vi "Periodic Tasks.vi"(8 "error in":errorcluster) -> ()   [LabVIEW 2018]
doc: "This VI runs in parallel to other tasks. It can contain as many user-defined periodic loops as you need. These can carry out PID or other sorts of timed response."
uses:
  <vilib>/Rock Robotics/WPI/Solenoid/WPI_SolenoidValue.ctl
  Phoenix-LabVIEW/Motor Controller/Controls/CTRE_Phoenix_MotorControl_ControlMode.ctl
  <vilib>/Rock Robotics/WPI/Utilities/WPI_GetSetVariantRefNum.vi
  <vilib>/Rock Robotics/WPI/Solenoid/WPI_SolenoidSetEnum.vi
  Global 1.vi
  <vilib>/Rock Robotics/Network Tables/NT Write Boolean.vi
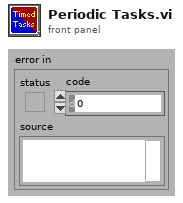
[diagram p1: front panel]
types:
  T1 = typedef "WPI_JoystickDevRef.ctl" = cluster{"Device":T2}
  T2 = typedef "WPI_JoystickDeviceEnum.ctl" = enum16{"USB 0", "USB 1", "USB 2", "USB 3", "USB 4", "USB 5"}
  T3 = typedef "WPI_RobotDriveDevRef.ctl" = cluster{"DevStatus":errorcluster, "Motors[]":T4[], "Square Inputs":bool, "Max Output":dbl}
  T4 = typedef "WPI_MotorControlDeviceRef.ctl" = cluster{"DeviceStatus":errorcluster, "Type":T5, "PWM":cluster{"PWM Channel":T6, "DeadBand":T7}, "CAN":cluster{"Device Number":u8, "SetOutput VI Ref":variant, "GetOutput VI Ref":variant, "Enable VI Ref":variant, "Disable VI Ref":variant, "Data":variant}, "Invert":bool, "DIO PWM":cluster{"PWM \"Enable\" Channel":T6, "DIOChannel":T8, "PWM Rate":dbl}}
  T5 = typedef "WPI_MotorControlType.ctl" = enum16{"PWM", "CAN", "DIO PWM"}
  T6 = typedef "FPGA_DIOPWMChannel.ctl" = enum8{"PWM 0", "PWM 1", "PWM 2", "PWM 3", "PWM 4", "PWM 5", "PWM 6", "PWM 7", "PWM 8", "PWM 9", "PWM MXP 0", "PWM MXP 1", "PWM MXP 2", "PWM MXP 3", "PWM MXP 4", "PWM MXP 5", "PWM MXP 6", "PWM MXP 7", "PWM MXP 8", "PWM MXP 9", "Invalid"}
  T7 = typedef "WPI_PWMDeadband.ctl" = cluster{"Name":string, "maxPositivePwm":i32, "minPositivePwm":i32, "centerPwm":i32, "maxNegativePwm":i32, "minNegativePwm":i32, "angularRange":u16}
  T8 = typedef "FPGA_DIOChannel.ctl" = enum8{"DIO 0", "DIO 1", "DIO 2", "DIO 3", "DIO 4", "DIO 5", "DIO 6", "DIO 7", "DIO 8", "DIO 9", "DIO MXP 0", "DIO MXP 1", "DIO MXP 2", "DIO MXP 3", "DIO MXP 4", "DIO MXP 5", "DIO MXP 6", "DIO MXP 7", "DIO MXP 8", "DIO MXP 9", "DIO MXP 10", "DIO MXP 11", "DIO MXP 12", "DIO MXP 13", "DIO MXP 14", "DIO MXP 15", "SPI Port CS1", "SPI Port CS2", "SPI Port CS3", "SPI Port MISO", "SPI Port MOSI", "Invalid"}
  T9 = cluster{"JoystickDevRef":T1, "RobotDriveDevRef":T3}
  T10 = typedef "WPI_SolenoidDevRef.ctl" = cluster{"DevStatus":errorcluster, "Pneumatics Control Module":u8, "Forward Solenoid Channel":T11, "Reverse Solenoid Channel":T11}
  T11 = typedef "WPI_SolenoidChannel.ctl" = enum8{"Solenoid 0", "Solenoid 1", "Solenoid 2", "Solenoid 3", "Solenoid 4", "Solenoid 5", "Solenoid 6", "Solenoid 7", "Invalid"}
  T12 = typedef "WPI_SolenoidValue.ctl" = enum16{"Off", "On", "Forward", "Reverse"}
  T13 = typedef "WPI_SwitchDevRef.ctl" = cluster{"DevStatus":errorcluster, "DIO Channel":T8, "CntIndex":T14, "Normally Closed":bool}
  T14 = typedef "FPGA_CounterCtrSystemIndex.ctl" = enum8{"Ctr 0", "Ctr 1", "Ctr 2", "Ctr 3", "Ctr 4", "Ctr 5", "Ctr 6", "Ctr 7", "Invalid"}
  T15 = typedef "CTRE_Phoenix_MotorControl_ControlMode.ctl" = u16
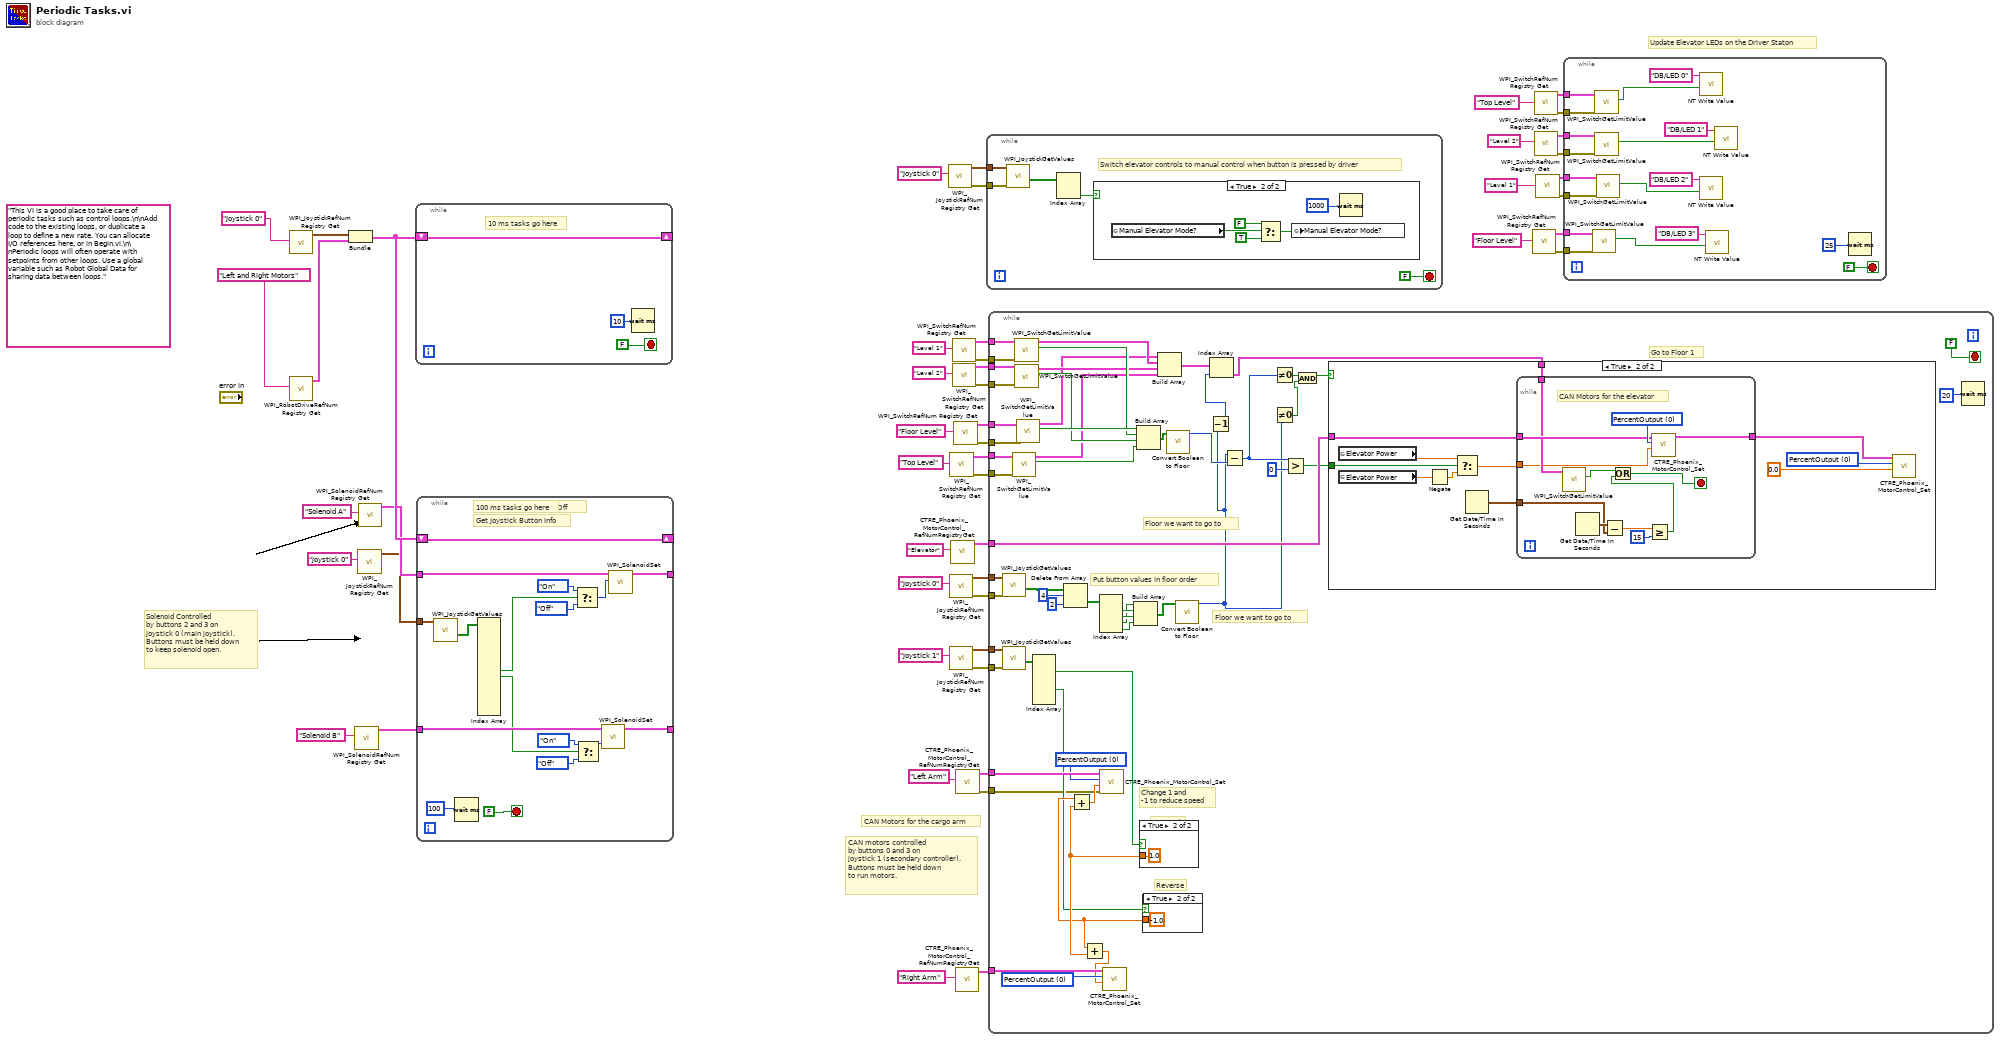
[diagram p0: block diagram]
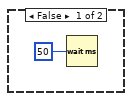
[diagram p2: hidden frame]
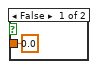
[diagram p3: hidden frame]
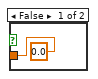
[diagram p4: hidden frame]
diagram:
  (unwired) "This VI is a good place to take care of periodic tasks such as control loops.\n\nAdd code to the existing loops, or duplicate a loop to define a new rate. You can allocate I/O references here, or in Begin.vi.\n\nPeriodic loops will often operate with setpoints from other loops. Use a global variable such as Robot Global Data for sharing data between loops."
  # "Update Elevator LEDs on the Driver Staton"
  # "CAN Motors for the cargo arm"
  # "CAN motors controlled\nby buttons 0 and 3 on \njoystick 1 (secondary controller).\nButtons must be held down\nto run motors."
  # "Solenoid Controlled\nby buttons 2 and 3 on \njoystick 0 (main joystick).\nButtons must be held down\nto keep solenoid open."
  n1 = call <vilib>:"WPI_JoystickRefNum Registry Get.vi"("refnum name"="Joystick 0") -> ("JoystickDevRef"=w49:T1)  [unwired: 1 in, 9 out]
  n2 = call <vilib>:"WPI_RobotDriveRefNum Registry Get.vi"("refnum name"="Left and Right Motors") -> ("RobotDriveDevRef"=w48:T3)  [unwired: 1 in, 9 out]
  n3 = Bundle("JoystickDevRef"=w49, "RobotDriveDevRef"=w48) -> (w47:T9)  [unwired: 1 out]
  n4 = call <vilib>:"WPI_SolenoidRefNum Registry Get.vi"("refnum name"="Solenoid B") -> ("SolenoidDevRef"=w39:T10)  [unwired: 9 in, 1 out]
  n5 = call <vilib>:"WPI_JoystickRefNum Registry Get.vi"("refnum name"="Joystick 0") -> ("JoystickDevRef"=w36:T1)  [unwired: 9 in, 1 out]
  n6 = call <vilib>:"WPI_SolenoidRefNum Registry Get.vi"("refnum name"="Solenoid A") -> ("SolenoidDevRef"=w40:T10)  [unwired: 9 in, 1 out]
  n7 = while {
    shift-right: [w52] -> _
    shift-left: w47 -> [w52]
    stop <- FALSE stop-if-true
    # "10 ms tasks go here"
    n8 = Wait (ms)(milliseconds to wait=u32 10) -> ()  [unwired: 1 out]
  }
  n9 = while {
    shift-right: [w69] -> _
    shift-left: w47 -> [w69]
    tunnel: w40 -> [w62]
    tunnel: w39 -> [w61]
    tunnel: [w60] -> _
    tunnel: [w59] -> _
    tunnel: w36 -> [w58]
    stop <- FALSE stop-if-true
    # "Get Joystick Button Info"
    # "Turn the solenoid On or Off"
    # "100 ms tasks go here"
    n10 = call <vilib>:"WPI_JoystickGetValues.vi"("JoystickDevRef"=w58) -> ("Buttons"=w57:bool[])  [unwired: 6 in, 4 out]
    n11 = Wait (ms)(milliseconds to wait=u32 100) -> ()  [unwired: 1 out]
    n12 = Index Array(array=w57) -> (element #7=w56:bool, element #8=w55:bool)  [unwired: 14 in, 12 out]
    n13 = Select(t=WPI_SolenoidValue."On" ("Value"), s=w56, f=WPI_SolenoidValue."Off" ("Value")) -> (s? t:f=w66:T12)
    n14 = Select(t=WPI_SolenoidValue."On" ("Value"), s=w55, f=WPI_SolenoidValue."Off" ("Value")) -> (s? t:f=w63:T12)
    n15 = call-poly <vilib>:"WPI_SolenoidSet.vi"("Value"=w63, "SolenoidDevRef"=w61) -> ("SolenoidDevRef"=w59:T10)  [unwired: 1 in, 8 out]
    n16 = call-poly <vilib>:"WPI_SolenoidSet.vi"("Value"=w66, "SolenoidDevRef"=w62) -> ("SolenoidDevRef"=w60:T10)  [unwired: 1 in, 8 out]
  }
  n17 = call <vilib>:"WPI_JoystickRefNum Registry Get.vi"("refnum name"="Joystick 0") -> ("error out"=w20:errorcluster, "JoystickDevRef"=w21:T1)  [unwired: 9 in]
  n18 = call <vilib>:"WPI_JoystickRefNum Registry Get.vi"("refnum name"="Joystick 0") -> ("error out"=w14:errorcluster, "JoystickDevRef"=w27:T1)  [unwired: 9 in]
  n19 = call <vilib>:"WPI_JoystickRefNum Registry Get.vi"("refnum name"="Joystick 1") -> ("error out"=w19:errorcluster, "JoystickDevRef"=w31:T1)  [unwired: 9 in]
  n20 = call <vilib>:"WPI_SwitchRefNum Registry Get.vi"("refnum name"="Top Level") -> ("error out"=w18:errorcluster, "SwitchDevRef"=w32:T13)  [unwired: 9 in]
  n21 = call "CTRE_Phoenix_MotorControl_RefNumRegistryGet.vi"("refnum name"="Elevator") -> ("PhoenixMotorControlDevRef"=w29:T4)  [unwired: 9 in, 1 out]
  n22 = call <vilib>:"WPI_SwitchRefNum Registry Get.vi"("refnum name"="Level 1") -> ("error out"=w15:errorcluster, "SwitchDevRef"=w43:T13)  [unwired: 9 in]
  n23 = call <vilib>:"WPI_SwitchRefNum Registry Get.vi"("refnum name"="Level 2") -> ("error out"=w16:errorcluster, "SwitchDevRef"=w42:T13)  [unwired: 9 in]
  n24 = call <vilib>:"WPI_SwitchRefNum Registry Get.vi"("refnum name"="Floor Level") -> ("error out"=w17:errorcluster, "SwitchDevRef"=w26:T13)  [unwired: 9 in]
  n25 = call "CTRE_Phoenix_MotorControl_RefNumRegistryGet.vi"("refnum name"="Right Arm") -> ("PhoenixMotorControlDevRef"=w34:T4)  [unwired: 9 in, 1 out]
  n26 = call "CTRE_Phoenix_MotorControl_RefNumRegistryGet.vi"("refnum name"="Left Arm") -> ("error out"=w13:errorcluster, "PhoenixMotorControlDevRef"=w35:T4)  [unwired: 9 in]
  n27 = while {
    tunnel: w21 -> [w76]
    tunnel: w20 -> [w75]
    stop <- FALSE stop-if-true
    # "Switch elevator controls to manual control when button is pressed by driver"
    n28 = call <vilib>:"WPI_JoystickGetValues.vi"("error in (no error)"=w75, "JoystickDevRef"=w76) -> ("Buttons"=w74:bool[])  [unwired: 5 in, 4 out]
    n29 = Index Array(array=w74) -> (element #2=w73:bool)  [unwired: 2 in, 1 out]
    n30 = case shown="True" w73 {
      frame False {
        n31 = Wait (ms)(milliseconds to wait=u32 50) -> ()  [unwired: 1 out]
      }
      frame True {
        n32 = global read "Global 1.vi" "Manual Elevator Mode?"() -> (w82:bool)
        n33 = Select(t=FALSE, s=w82, f=TRUE) -> (s? t:f=w81:bool)
        n34 = global write "Global 1.vi" "Manual Elevator Mode?"(w81) -> ()
        n35 = Wait (ms)(milliseconds to wait=u32 1000) -> ()  [unwired: 1 out]
      }
    }
  }
  n36 = while {
    tunnel: w43 -> [w136]
    tunnel: w42 -> [w135]
    tunnel: w35 -> [w134]
    tunnel: w34 -> [w133]
    tunnel: w32 -> [w132]
    tunnel: w31 -> [w131]
    tunnel: w29 -> [w128]
    tunnel: w27 -> [w130]
    tunnel: w26 -> [w129]
    tunnel: w19 -> [w89]
    tunnel: w18 -> [w88]
    tunnel: w17 -> [w87]
    tunnel: w16 -> [w86]
    tunnel: w15 -> [w85]
    tunnel: w14 -> [w84]
    tunnel: w13 -> [w83]
    stop <- FALSE stop-if-true
    w97 = T15 0 items=["PercentOutput"=0, "Position"=1, "Velocity"=2, "Current"=3, "Follower"=5, "MotionProfile"=6, "MotionMagic"=7, "MotionProfileArc"=10, "Disabled"=15] ("Control Mode")
    w99 = T15 0 items=["PercentOutput"=0, "Position"=1, "Velocity"=2, "Current"=3, "Follower"=5, "MotionProfile"=6, "MotionMagic"=7, "MotionProfileArc"=10, "Disabled"=15] ("Control Mode")
    # "Change 1 and\n-1 to reduce speed"
    # "Forward"
    # "Reverse"
    # "Put button values in floor order"
    # "Floor we want to go to"
    # "Floor we want to go to"
    # "Go to Floor 1"
    n37 = call <vilib>:"WPI_JoystickGetValues.vi"("error in (no error)"=w84, "JoystickDevRef"=w130) -> ("Buttons"=w90:bool[])  [unwired: 5 in, 4 out]
    n38 = call <vilib>:"WPI_JoystickGetValues.vi"("error in (no error)"=w89, "JoystickDevRef"=w131) -> ("Buttons"=w94:bool[])  [unwired: 5 in, 4 out]
    n39 = call <vilib>:"WPI_SwitchGetLimitValue.vi"("error in (no error)"=w88, "SwitchDevRef"=w132) -> ("Switch Pressed"=w124:bool, "SwitchDevRef"=w107:T13)  [unwired: 7 in, 1 out]
    n40 = call <vilib>:"WPI_SwitchGetLimitValue.vi"("error in (no error)"=w85, "SwitchDevRef"=w136) -> ("Switch Pressed"=w116:bool, "SwitchDevRef"=w109:T13)  [unwired: 7 in, 1 out]
    n41 = call <vilib>:"WPI_SwitchGetLimitValue.vi"("error in (no error)"=w86, "SwitchDevRef"=w135) -> ("Switch Pressed"=w115:bool, "SwitchDevRef"=w108:T13)  [unwired: 7 in, 1 out]
    n42 = call <vilib>:"WPI_SwitchGetLimitValue.vi"("error in (no error)"=w87, "SwitchDevRef"=w129) -> ("Switch Pressed"=w123:bool, "SwitchDevRef"=w106:T13)  [unwired: 7 in, 1 out]
    n43 = Index Array(array=w94) -> (element #1=w92:bool, element #4=w91:bool)  [unwired: 6 in, 4 out]
    n44 = Delete From Array(array=w90, length=4, index=2) -> (deleted portion=w122:bool[])  [unwired: 1 out]
    n45 = Index Array(array=w122) -> (element #1=w121:bool, element #2=w120:bool, element #3=w119:bool, element #4=w118:bool)  [unwired: 4 in]
    n46 = Build Array(w119, w121, w120, w118) -> (w117:bool[])
    n47 = Build Array(w123, w116, w115, w124) -> (w125:bool[])
    n48 = case shown="True" w92 {
      tunnel: [0.0 1.0] -> w95
      frame False {
      }
      frame True {
      }
    }
    n49 = case shown="True" w91 {
      tunnel: [0.0 -1.0] -> w93
      frame False {
      }
      frame True {
      }
    }
    n50 = Add(x=w93, y=w95) -> (x+y=w98:dbl)
    n51 = Add(x=w93, y=w95) -> (x+y=w96:dbl)
    n52 = call "CTRE_Phoenix_MotorControl_Set.vi"("error in (no error)"=w83, "Output"=w98, "Control Mode"=w99, "PhoenixMotorControlDevRef"=w134) -> ()  [unwired: 6 in, 2 out]
    n53 = call "CTRE_Phoenix_MotorControl_Set.vi"("Output"=w96, "Control Mode"=w97, "PhoenixMotorControlDevRef"=w133) -> ()  [unwired: 7 in, 2 out]
    n54 = Build Array(w106, w109, w108, w107) -> (w105:T13[])
    n55 = call "Convert Boolean to Floor.vi"("Boolean array"=w125) -> ("Floor Number"=w113:i32)  [unwired: 8 in, 2 out]
    n56 = call "Convert Boolean to Floor.vi"("Boolean array"=w117) -> ("Floor Number"=w101:i32)  [unwired: 8 in, 2 out]
    n57 = Decrement(x=w101) -> (x-1=w103:i32)
    n58 = Index Array(array=w105, index=w103) -> (element=w104:T13)
    n59 = Subtract(x=w101, y=w113) -> (x-y=w112:i32)
    n60 = Not Equal To 0?(x=w112) -> (x != 0?=w114:bool)
    n61 = Not Equal To 0?(x=w101) -> (x != 0?=w100:bool)
    n62 = Greater?(x=w112, y=0) -> (0:w110:bool)
    n63 = And(x=w114, y=w100) -> (x .and. y?=w102:bool)
    n64 = case shown="True" w102 {
      tunnel: w128 -> [_ w153]
      tunnel: w104 -> [_ w149]
      tunnel: w110 -> [_ w146]
      frame False {
      }
      frame True {
        w152 = T15 0 items=["PercentOutput"=0, "Position"=1, "Velocity"=2, "Current"=3, "Follower"=5, "MotionProfile"=6, "MotionMagic"=7, "MotionProfileArc"=10, "Disabled"=15] ("Control Mode")
        n65 = global read "Global 1.vi" "Elevator Power"() -> (w145:dbl)
        n66 = global read "Global 1.vi" "Elevator Power"() -> (w143:dbl)
        n67 = Negate(x=w143) -> (-x=w144:dbl)
        n68 = Select(t=w145, s=w146, f=w144) -> (s? t:f=w148:dbl)
        n69 = Get Date/Time In Seconds() -> (seconds since 1Jan1904=w147:timestamp)
        n70 = while {
          tunnel: w153 -> [w164]
          tunnel: [w163] -> w150
          tunnel: w149 -> [w162]
          tunnel: w148 -> [w161]
          tunnel: w147 -> [w157]
          stop <- w160 stop-if-true
          w165 = T15 0 items=["PercentOutput"=0, "Position"=1, "Velocity"=2, "Current"=3, "Follower"=5, "MotionProfile"=6, "MotionMagic"=7, "MotionProfileArc"=10, "Disabled"=15] ("Control Mode")
          # "CAN Motors for the elevator"
          n71 = call <vilib>:"WPI_SwitchGetLimitValue.vi"("SwitchDevRef"=w162) -> ("Switch Pressed"=w159:bool)  [unwired: 8 in, 2 out]
          n72 = Get Date/Time In Seconds() -> (seconds since 1Jan1904=w158:timestamp)
          n73 = Subtract(x=w158, y=w157) -> (x-y=w155:dbl)
          n74 = Greater Or Equal?(x=w155, y=15) -> (x >= y?=w154:bool)
          n75 = Or(x=w159, y=w154) -> (x .or. y?=w160:bool)
          n76 = call "CTRE_Phoenix_MotorControl_Set.vi"("Output"=w161, "Control Mode"=w165, "PhoenixMotorControlDevRef"=w164) -> ("PhoenixMotorControlDevRef"=w163:T4)  [unwired: 7 in, 1 out]
        }
        n77 = call "CTRE_Phoenix_MotorControl_Set.vi"("Output"=0.0, "Control Mode"=w152, "PhoenixMotorControlDevRef"=w150) -> ()  [unwired: 7 in, 2 out]
      }
    }
    n78 = Wait (ms)(milliseconds to wait=u32 20) -> ()  [unwired: 1 out]
  }
  n79 = call <vilib>:"WPI_SwitchRefNum Registry Get.vi"("refnum name"="Floor Level") -> ("error out"=w7:errorcluster, "SwitchDevRef"=w6:T13)  [unwired: 9 in]
  n80 = call <vilib>:"WPI_SwitchRefNum Registry Get.vi"("refnum name"="Top Level") -> ("error out"=w11:errorcluster, "SwitchDevRef"=w12:T13)  [unwired: 9 in]
  n81 = call <vilib>:"WPI_SwitchRefNum Registry Get.vi"("refnum name"="Level 2") -> ("error out"=w9:errorcluster, "SwitchDevRef"=w10:T13)  [unwired: 9 in]
  n82 = call <vilib>:"WPI_SwitchRefNum Registry Get.vi"("refnum name"="Level 1") -> ("error out"=w5:errorcluster, "SwitchDevRef"=w8:T13)  [unwired: 9 in]
  n83 = while {
    tunnel: w12 -> [w183]
    tunnel: w11 -> [w182]
    tunnel: w10 -> [w181]
    tunnel: w9 -> [w180]
    tunnel: w8 -> [w179]
    tunnel: w7 -> [w178]
    tunnel: w6 -> [w177]
    tunnel: w5 -> [w176]
    stop <- FALSE stop-if-true
    n84 = call <vilib>:"WPI_SwitchGetLimitValue.vi"("error in (no error)"=w178, "SwitchDevRef"=w177) -> ("Switch Pressed"=w168:bool)  [unwired: 7 in, 2 out]
    n85 = call <vilib>:"WPI_SwitchGetLimitValue.vi"("error in (no error)"=w182, "SwitchDevRef"=w183) -> ("Switch Pressed"=w174:bool)  [unwired: 7 in, 2 out]
    n86 = call <vilib>:"WPI_SwitchGetLimitValue.vi"("error in (no error)"=w180, "SwitchDevRef"=w181) -> ("Switch Pressed"=w172:bool)  [unwired: 7 in, 2 out]
    n87 = call <vilib>:"WPI_SwitchGetLimitValue.vi"("error in (no error)"=w176, "SwitchDevRef"=w179) -> ("Switch Pressed"=w170:bool)  [unwired: 7 in, 2 out]
    n88 = call-poly <vilib>:"NT Write Value.vi"("Boolean"=w174, "Name"="DB/LED 0") -> ()  [unwired: 9 in, 1 out]
    n89 = call-poly <vilib>:"NT Write Value.vi"("Boolean"=w170, "Name"="DB/LED 2") -> ()  [unwired: 9 in, 1 out]
    n90 = call-poly <vilib>:"NT Write Value.vi"("Boolean"=w168, "Name"="DB/LED 3") -> ()  [unwired: 9 in, 1 out]
    n91 = call-poly <vilib>:"NT Write Value.vi"("Boolean"=w172, "Name"="DB/LED 1") -> ()  [unwired: 9 in, 1 out]
    n92 = Wait (ms)(milliseconds to wait=u32 25 ("millisecond timer value")) -> ()  [unwired: 1 out]
  }
